vi "Pneumatic box control.vi"() -> ()   [LabVIEW 2018]
panel:
  out "出口气压":dbl(graph)
  out "x-y":u32
  out "错误输出 2":errorcluster caption="错误输出"
  out "手动给定值 4":dbl
  out "手动给定值 3":dbl
  out "手动给定值 2":dbl
  out "手动给定值":dbl
  in  "自动":bool=TRUE
  out "低负测量值":dbl
  out "低负给定值":dbl
  out "低正测量值":dbl
  out "低正给定值":dbl
  out "高负测量值":dbl
  out "高负给定值":dbl
  out "高正给定值":dbl
  out "高正测量值":dbl
  out "低负气压/psi":cluster{dbl, "低负":sgl}(graph)
  out "低正气压/psi":cluster{dbl, "低正":sgl}(graph)
  out "高负气压/psi":cluster{dbl, "高负":sgl}(graph)
  out "高正气压/psi":cluster{"高正":sgl, sgl}(graph)
  out "错误输出":errorcluster
  in  "case":dbl
  in  "停止":bool
  in  "低负":sgl(knob)=-0.22290154
  in  "高负":sgl(knob)=-1.1416342
  in  "低正":sgl(knob)=0.7104824 scale=0.0..2.0
  in  "高正":sgl(knob)=15.0 scale=0.0..15.0
  in  "低负开关":bool
  in  "低正开关":bool
  in  "大气压":bool
  in  "高负开关":bool
  in  "高正开关":bool
  in  "采样率":u32=255
  in  "DevIndex":i32
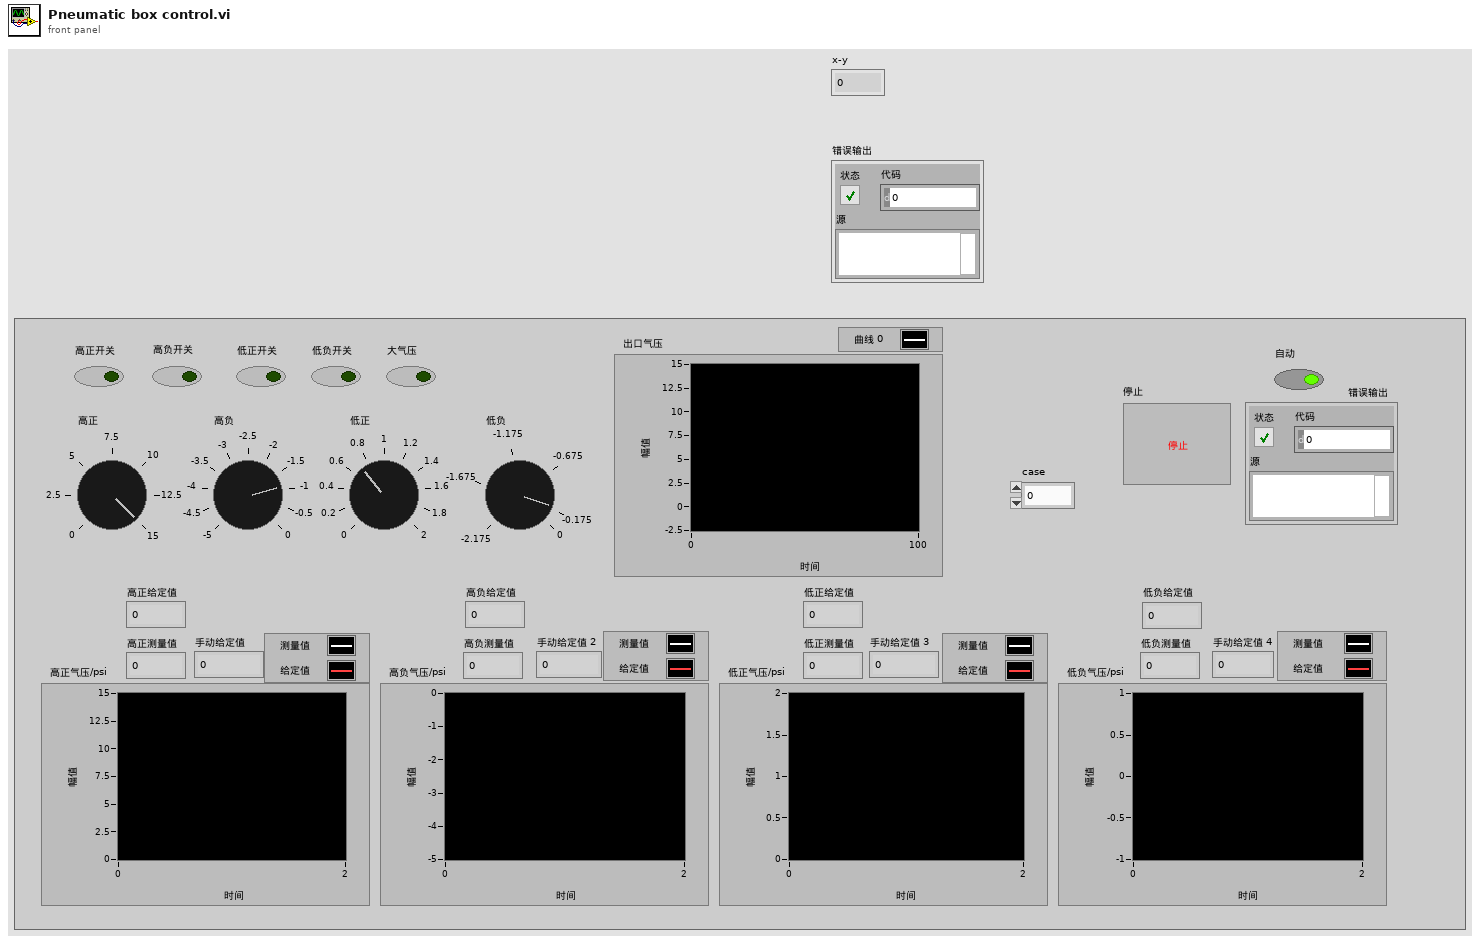
[diagram p1: front panel]
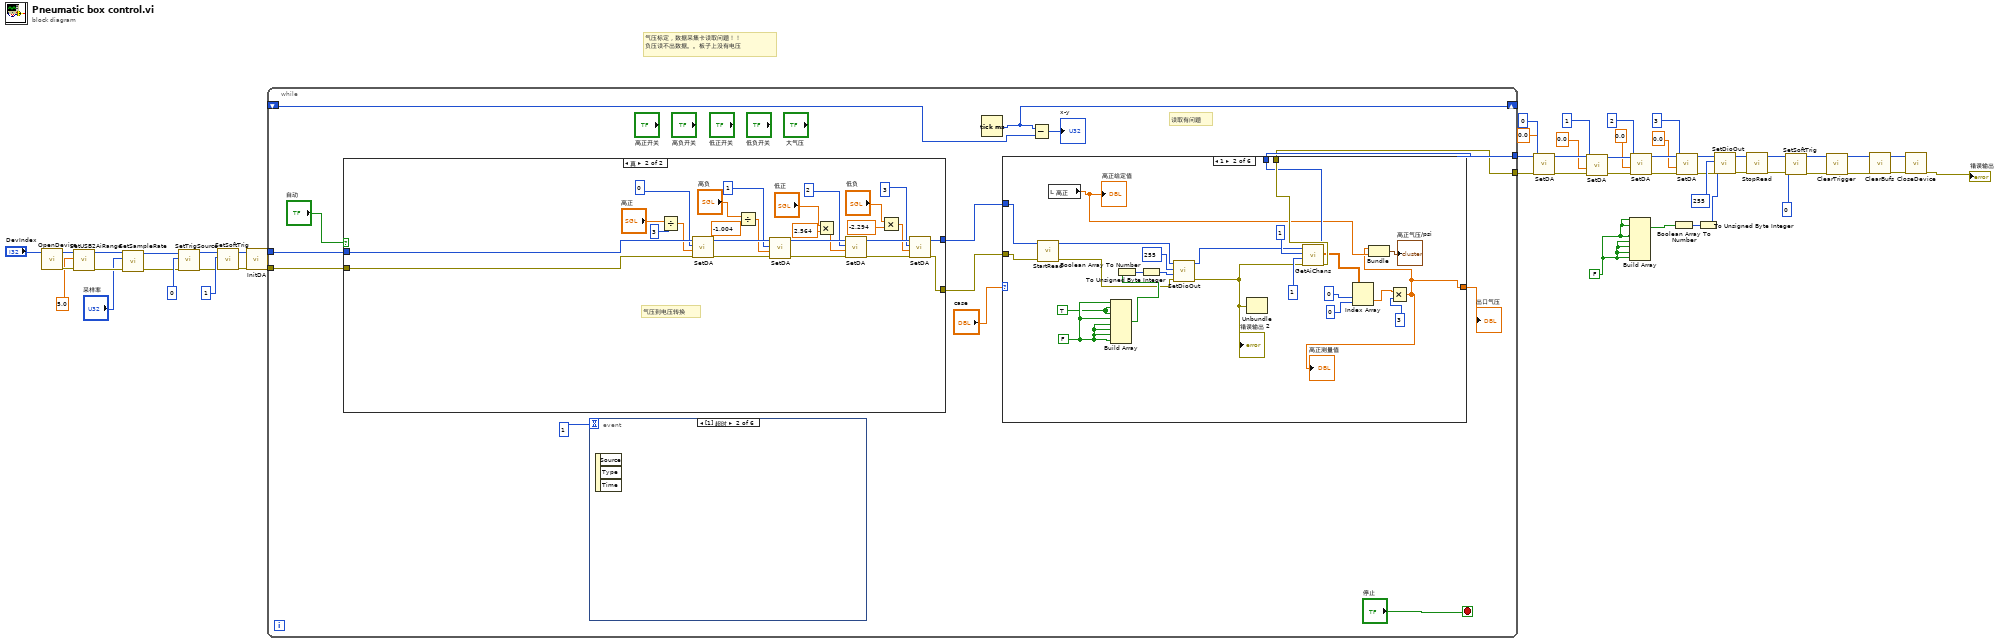
[diagram p0: block diagram]
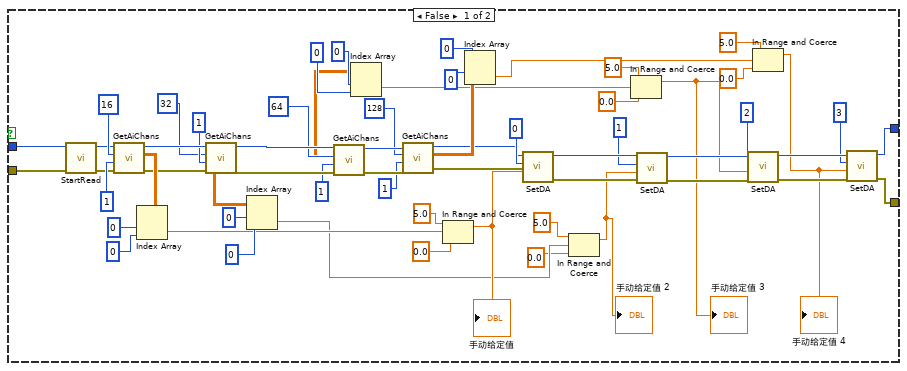
[diagram p2: hidden frame]
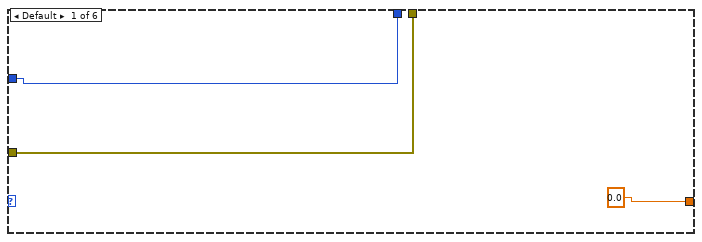
[diagram p3: hidden frame]
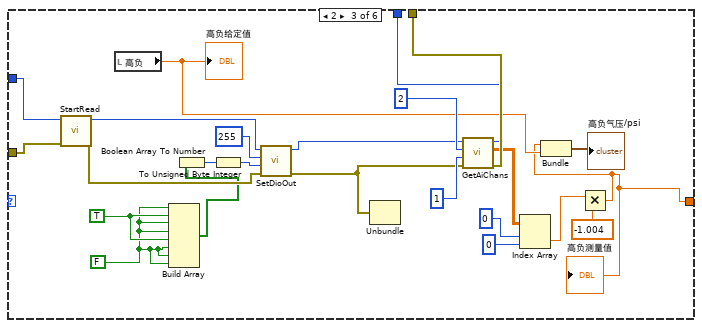
[diagram p4: hidden frame]
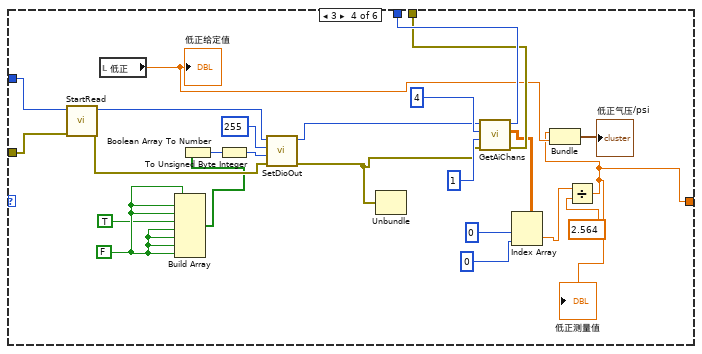
[diagram p5: hidden frame]
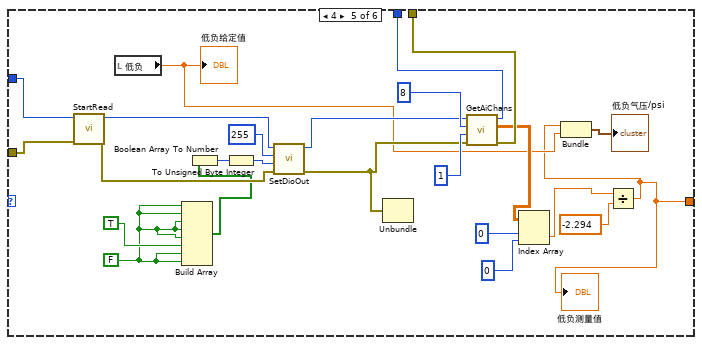
[diagram p6: hidden frame]
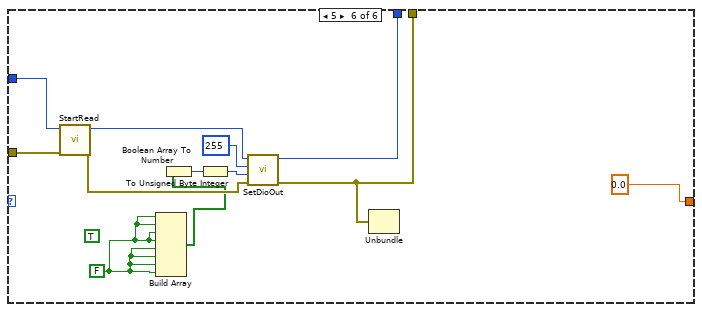
[diagram p7: hidden frame]
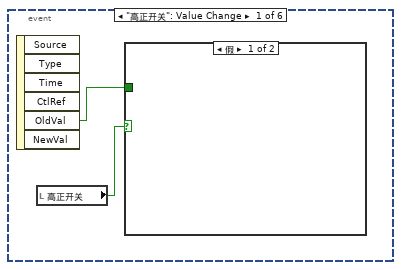
[diagram p8: hidden frame]
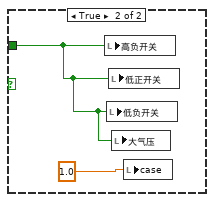
[diagram p9: hidden frame]
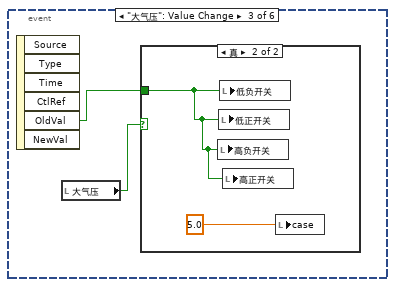
[diagram p10: hidden frame]
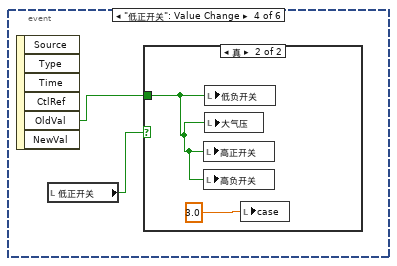
[diagram p12: hidden frame]
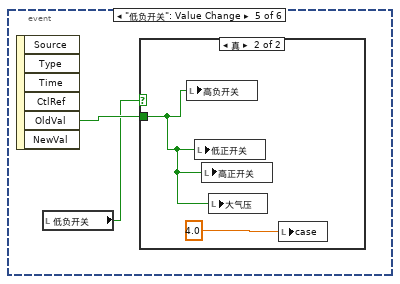
[diagram p14: hidden frame]
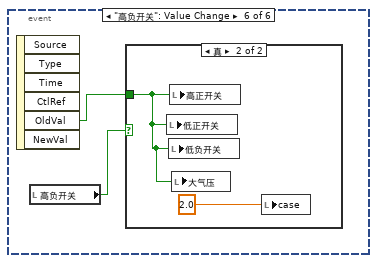
[diagram p16: hidden frame]
diagram:
  w9 = FALSE
  # "气压标定，数据采集卡读取问题！！\n负压读不出数据。。板子上没有电压"
  n1 = call "OpenDevice.vi"("DevIndex"="DevIndex") -> ("错误输出"=w44:errorcluster, "DevIndex Output"=w46:i32)  [unwired: 9 in]
  n2 = call "SetUSB2AiRange.vi"("错误输入（无错误）"=w44, "Range"=sgl 5.0, "DevIndex"=w46) -> ("错误输出"=w35:errorcluster, "DevIndex Output"=w37:i32)  [unwired: 7 in]
  n3 = call "SetSampleRate.vi"("错误输入（无错误）"=w35, "SampleRate"="采样率", "DevIndex"=w37) -> ("错误输出"=w34:errorcluster, "DevIndex Output"=w36:i32)  [unwired: 7 in]
  n4 = call "SetTrigSource.vi"("错误输入（无错误）"=w34, "TrigSource"=u8 0, "DevIndex"=w36) -> ("错误输出"=w39:errorcluster, "DevIndex Output"=w40:i32)  [unwired: 7 in]
  n5 = call "SetSoftTrig.vi"("错误输入（无错误）"=w39, "Trig"=u8 1, "DevIndex"=w40) -> ("错误输出"=w43:errorcluster, "DevIndex Output"=w45:i32)  [unwired: 7 in]
  n6 = call "InitDA.vi"("错误输入（无错误）"=w43, "DevIndex"=w45) -> ("错误输出"=w50:errorcluster, "DevIndex Output"=w51:i32)  [unwired: 8 in]
  n7 = while {
    tunnel: w51 -> [w65]
    tunnel: w50 -> [w64]
    tunnel: [w57] -> w11
    tunnel: [w56] -> w10
    shift-right: [w55] -> _
    shift-left: _ -> [w54]
    stop <- "停止" stop-if-true
    # "读取有问题"
    n8 = case shown="真" "自动" {
      tunnel: w65 -> [w116 w146]
      tunnel: w64 -> [w117 w145]
      tunnel: [w86 w141] -> w63
      tunnel: [w85 w140] -> w62
      frame False {
        n9 = call "StartRead.vi"("错误输入（无错误）"=w117, "DevIndex"=w116) -> ("错误输出"=w112:errorcluster, "DevIndex Output"=w114:i32)  [unwired: 8 in]
        n10 = call "GetAiChans.vi"("错误输入（无错误）"=w112, "Num"=u32 1, "ChanSel"=u16 16, "DevIndex"=w114) -> ("错误输出"=w102:errorcluster, "Ai"=w111:sgl[][], "DevIndex Output"=w103:i32)  [unwired: 4 in, 1 out]
        n11 = Index Array(array=w111, index (row)=0, index (col)=0) -> (element=w79:sgl)
        n12 = call "GetAiChans.vi"("错误输入（无错误）"=w102, "Num"=u32 1, "ChanSel"=u16 32, "DevIndex"=w103) -> ("错误输出"=w98:errorcluster, "Ai"=w108:sgl[][], "DevIndex Output"=w99:i32)  [unwired: 4 in, 1 out]
        n13 = Index Array(array=w108, index (row)=0, index (col)=0) -> (element=w78:sgl)
        n14 = call "GetAiChans.vi"("错误输入（无错误）"=w98, "Num"=u32 1, "ChanSel"=u16 64, "DevIndex"=w99) -> ("错误输出"=w93:errorcluster, "Ai"=w95:sgl[][], "DevIndex Output"=w94:i32)  [unwired: 4 in, 1 out]
        n15 = Index Array(array=w95, index (row)=0, index (col)=0) -> (element=w69:sgl)
        n16 = call "GetAiChans.vi"("错误输入（无错误）"=w93, "Num"=u32 1, "ChanSel"=u16 128, "DevIndex"=w94) -> ("错误输出"=w83:errorcluster, "Ai"=w90:sgl[][], "DevIndex Output"=w84:i32)  [unwired: 4 in, 1 out]
        n17 = In Range and Coerce(upper limit=5.0, x=w79, lower limit=0.0) -> (coerced(x)=w80:dbl)  [unwired: 1 out]
        "手动给定值" <- w80
        n18 = Index Array(array=w90, index (row)=0, index (col)=0) -> (element=w71:sgl)
        n19 = call "SetDA.vi"("错误输入（无错误）"=w83, "DAVolt"=w80, "DANum"=u8 0, "DevIndex"=w84) -> ("错误输出"=w125:errorcluster, "DevIndex Output"=w126:i32)  [unwired: 6 in]
        n20 = In Range and Coerce(upper limit=5.0, x=w78, lower limit=0.0) -> (coerced(x)=w67:dbl)  [unwired: 1 out]
        "手动给定值 2" <- w67
        n21 = In Range and Coerce(upper limit=5.0, x=w69, lower limit=0.0) -> (coerced(x)=w68:dbl)  [unwired: 1 out]
        "手动给定值 3" <- w68
        n22 = call "SetDA.vi"("错误输入（无错误）"=w125, "DAVolt"=w67, "DANum"=u8 1, "DevIndex"=w126) -> ("错误输出"=w124:errorcluster, "DevIndex Output"=w123:i32)  [unwired: 6 in]
        n23 = call "SetDA.vi"("错误输入（无错误）"=w124, "DAVolt"=w68, "DANum"=u8 2, "DevIndex"=w123) -> ("错误输出"=w121:errorcluster, "DevIndex Output"=w122:i32)  [unwired: 6 in]
        n24 = In Range and Coerce(upper limit=5.0, x=w71, lower limit=0.0) -> (coerced(x)=w70:dbl)  [unwired: 1 out]
        "手动给定值 4" <- w70
        n25 = call "SetDA.vi"("错误输入（无错误）"=w121, "DAVolt"=w70, "DANum"=u8 3, "DevIndex"=w122) -> ("错误输出"=w85:errorcluster, "DevIndex Output"=w86:i32)  [unwired: 6 in]
      }
      frame True {
        # "气压到电压转换"
        n26 = Divide(x="高正", y=3) -> (x/y=w130:sgl)
        n27 = call "SetDA.vi"("错误输入（无错误）"=w145, "DAVolt"=w130, "DANum"=u8 0, "DevIndex"=w146) -> ("错误输出"=w151:errorcluster, "DevIndex Output"=w152:i32)  [unwired: 6 in]
        n28 = Divide(x="高负", y=-1.004) -> (x/y=w128:dbl)
        n29 = call "SetDA.vi"("错误输入（无错误）"=w151, "DAVolt"=w128, "DANum"=u8 1, "DevIndex"=w152) -> ("错误输出"=w150:errorcluster, "DevIndex Output"=w149:i32)  [unwired: 6 in]
        n30 = Multiply(x="低正", y=2.564) -> (x*y=w129:dbl)
        n31 = call "SetDA.vi"("错误输入（无错误）"=w150, "DAVolt"=w129, "DANum"=u8 2, "DevIndex"=w149) -> ("错误输出"=w147:errorcluster, "DevIndex Output"=w148:i32)  [unwired: 6 in]
        n32 = Multiply(x="低负", y=-2.294) -> (x*y=w127:dbl)
        n33 = call "SetDA.vi"("错误输入（无错误）"=w147, "DAVolt"=w127, "DANum"=u8 3, "DevIndex"=w148) -> ("错误输出"=w140:errorcluster, "DevIndex Output"=w141:i32)  [unwired: 6 in]
      }
    }
    n34 = event shown="[1] 超时" {
      selector: _ -> [_ _ _ _ _ _]
      dyn-events: _ -> [_ _ _ _ _ _]
      timeout: 1 -> [_ _ _ _ _ _]
      event "高正开关": Value Change {
        n35 = event-data() -> ("OldVal"=w264:bool)  [unwired: 1 in, 5 out]
        n36 = local read "高正开关"() -> (w265:bool)
        n37 = case shown="假" w265 {
          tunnel: w264 -> [_ w267]
          frame False {
          }
          frame True {
            n38 = local write "高负开关"(w267) -> ()
            n39 = local write "低负开关"(w267) -> ()
            n40 = local write "低正开关"(w267) -> ()
            n41 = local write "大气压"(w267) -> ()
            n42 = local write "case"(1.0) -> ()
          }
        }
      }
      event Timeout {
        n43 = event-data() -> ()  [unwired: 1 in, 3 out]
      }
      event "大气压": Value Change {
        n44 = event-data() -> ("OldVal"=w268:bool)  [unwired: 1 in, 5 out]
        n45 = local read "大气压"() -> (w269:bool)
        n46 = case shown="真" w269 {
          tunnel: w268 -> [_ w271]
          frame False {
          }
          frame True {
            n47 = local write "高负开关"(w271) -> ()
            n48 = local write "低正开关"(w271) -> ()
            n49 = local write "低负开关"(w271) -> ()
            n50 = local write "高正开关"(w271) -> ()
            n51 = local write "case"(5.0) -> ()
          }
        }
      }
      event "低正开关": Value Change {
        n52 = event-data() -> ("OldVal"=w273:bool)  [unwired: 1 in, 5 out]
        n53 = local read "低正开关"() -> (w272:bool)
        n54 = case shown="真" w272 {
          tunnel: w273 -> [_ w275]
          frame False {
          }
          frame True {
            n55 = local write "高正开关"(w275) -> ()
            n56 = local write "高负开关"(w275) -> ()
            n57 = local write "低负开关"(w275) -> ()
            n58 = local write "大气压"(w275) -> ()
            n59 = local write "case"(3.0) -> ()
          }
        }
      }
      event "低负开关": Value Change {
        n60 = event-data() -> ("OldVal"=w277:bool)  [unwired: 1 in, 5 out]
        n61 = local read "低负开关"() -> (w276:bool)
        n62 = case shown="真" w276 {
          tunnel: w277 -> [_ w279]
          frame False {
          }
          frame True {
            n63 = local write "高负开关"(w279) -> ()
            n64 = local write "低正开关"(w279) -> ()
            n65 = local write "高正开关"(w279) -> ()
            n66 = local write "大气压"(w279) -> ()
            n67 = local write "case"(4.0) -> ()
          }
        }
      }
      event "高负开关": Value Change {
        n68 = event-data() -> ("OldVal"=w281:bool)  [unwired: 1 in, 5 out]
        n69 = local read "高负开关"() -> (w280:bool)
        n70 = case shown="真" w280 {
          tunnel: w281 -> [_ w283]
          frame False {
          }
          frame True {
            n71 = local write "低正开关"(w283) -> ()
            n72 = local write "低负开关"(w283) -> ()
            n73 = local write "高正开关"(w283) -> ()
            n74 = local write "大气压"(w283) -> ()
            n75 = local write "case"(2.0) -> ()
          }
        }
      }
    }
    n76 = Tick Count (ms)() -> (millisecond timer value=w55:u32)
    n77 = case shown="1" "case" {
      tunnel: w63 -> [w155 w175 w197 w221 w245 w257]
      tunnel: w62 -> [w154 w174 w196 w220 w244 w256]
      tunnel: [w155 w164 w188 w215 w237 w254] -> w57
      tunnel: [w154 w165 w189 w214 w238 w253] -> w56
      tunnel: [0.0 w156 w180 w206 w229 0.0] -> w60
      frame Default {
      }
      frame 1 {
        w172 = TRUE
        w173 = FALSE
        n78 = call "StartRead.vi"("错误输入（无错误）"=w174, "DevIndex"=w175) -> ("错误输出"=w170:errorcluster, "DevIndex Output"=w171:i32)  [unwired: 8 in]
        n79 = local read "高正"() -> (w159:sgl)
        "高正给定值" <- w159
        n80 = Build Array(w173, w172, w172, w173, w173, w173, w173, w173) -> (w176:bool[])
        n81 = Boolean Array To Number(Boolean array=w176) -> (number=w179:u32)
        n82 = To Unsigned Byte Integer(number=w179) -> (unsigned 8bit integer=w178:u8)
        n83 = call "SetDioOut.vi"("错误输入（无错误）"=w170, "DioOut"=w178, "DioChanSel"=u8 255, "DevIndex"=w171) -> ("错误输出"=w166:errorcluster, "DevIndex Output"=w167:i32)  [unwired: 6 in]
        "错误输出 2" <- w166
        n84 = Unbundle(w166) -> ()  [unwired: 3 out]
        n85 = call "GetAiChans.vi"("错误输入（无错误）"=w166, "Num"=u32 1, "ChanSel"=u16 1, "DevIndex"=w167) -> ("错误输出"=w165:errorcluster, "Ai"=w161:sgl[][], "DevIndex Output"=w164:i32)  [unwired: 4 in, 1 out]
        n86 = Index Array(array=w161, index (row)=0, index (col)=0) -> (element=w157:sgl)
        n87 = Multiply(x=w157, y=3) -> (x*y=w156:sgl)
        "高正测量值" <- w156
        n88 = Bundle(w156, "高正"=w159) -> (→"高正气压/psi":cluster{sgl, "高正":sgl})  [unwired: 1 in]
      }
      frame 2 {
        w195 = TRUE
        w194 = FALSE
        n89 = call "StartRead.vi"("错误输入（无错误）"=w196, "DevIndex"=w197) -> ("错误输出"=w199:errorcluster, "DevIndex Output"=w200:i32)  [unwired: 8 in]
        n90 = local read "高负"() -> (w184:sgl)
        "高负给定值" <- w184
        n91 = Build Array(w194, w195, w194, w194, w195, w194, w194, w194) -> (w198:bool[])
        n92 = Boolean Array To Number(Boolean array=w198) -> (number=w203:u32)
        n93 = To Unsigned Byte Integer(number=w203) -> (unsigned 8bit integer=w202:u8)
        n94 = call "SetDioOut.vi"("错误输入（无错误）"=w199, "DioOut"=w202, "DioChanSel"=u8 255, "DevIndex"=w200) -> ("错误输出"=w190:errorcluster, "DevIndex Output"=w191:i32)  [unwired: 6 in]
        n95 = Unbundle(w190) -> ()  [unwired: 3 out]
        n96 = call "GetAiChans.vi"("错误输入（无错误）"=w190, "Num"=u32 1, "ChanSel"=u16 2, "DevIndex"=w191) -> ("错误输出"=w189:errorcluster, "Ai"=w185:sgl[][], "DevIndex Output"=w188:i32)  [unwired: 4 in, 1 out]
        n97 = Index Array(array=w185, index (row)=0, index (col)=0) -> (element=w182:sgl)
        n98 = Multiply(x=w182, y=-1.004) -> (x*y=w180:dbl)
        "高负测量值" <- w180
        n99 = Bundle(w180, "高负"=w184) -> (→"高负气压/psi":cluster{dbl, "高负":sgl})  [unwired: 1 in]
      }
      frame 3 {
        w205 = FALSE
        n100 = call "StartRead.vi"("错误输入（无错误）"=w220, "DevIndex"=w221) -> ("错误输出"=w223:errorcluster, "DevIndex Output"=w224:i32)  [unwired: 8 in]
        n101 = local read "低正"() -> (w209:sgl)
        "低正给定值" <- w209
        n102 = Build Array(w205, w205, w205, TRUE, w205, w205, w205, w205) -> (w222:bool[])
        n103 = Boolean Array To Number(Boolean array=w222) -> (number=w227:u32)
        n104 = To Unsigned Byte Integer(number=w227) -> (unsigned 8bit integer=w226:u8)
        n105 = call "SetDioOut.vi"("错误输入（无错误）"=w223, "DioOut"=w226, "DioChanSel"=u8 255, "DevIndex"=w224) -> ("错误输出"=w216:errorcluster, "DevIndex Output"=w217:i32)  [unwired: 6 in]
        n106 = Unbundle(w216) -> ()  [unwired: 3 out]
        n107 = call "GetAiChans.vi"("错误输入（无错误）"=w216, "Num"=u32 1, "ChanSel"=u16 4, "DevIndex"=w217) -> ("错误输出"=w214:errorcluster, "Ai"=w211:sgl[][], "DevIndex Output"=w215:i32)  [unwired: 4 in, 1 out]
        n108 = Index Array(array=w211, index (row)=0, index (col)=0) -> (element=w208:sgl)
        n109 = Divide(x=w208, y=2.564) -> (x/y=w206:dbl)
        "低正测量值" <- w206
        n110 = Bundle(w206, "低正"=w209) -> (→"低正气压/psi":cluster{dbl, "低正":sgl})  [unwired: 1 in]
      }
      frame 4 {
        w228 = FALSE
        n111 = call "StartRead.vi"("错误输入（无错误）"=w244, "DevIndex"=w245) -> ("错误输出"=w247:errorcluster, "DevIndex Output"=w248:i32)  [unwired: 8 in]
        n112 = local read "低负"() -> (w233:sgl)
        "低负给定值" <- w233
        n113 = Build Array(w228, w228, w228, w228, w228, TRUE, w228, w228) -> (w246:bool[])
        n114 = Boolean Array To Number(Boolean array=w246) -> (number=w251:u32)
        n115 = To Unsigned Byte Integer(number=w251) -> (unsigned 8bit integer=w250:u8)
        n116 = call "SetDioOut.vi"("错误输入（无错误）"=w247, "DioOut"=w250, "DioChanSel"=u8 255, "DevIndex"=w248) -> ("错误输出"=w239:errorcluster, "DevIndex Output"=w240:i32)  [unwired: 6 in]
        n117 = Unbundle(w239) -> ()  [unwired: 3 out]
        n118 = call "GetAiChans.vi"("错误输入（无错误）"=w239, "Num"=u32 1, "ChanSel"=u16 8, "DevIndex"=w240) -> ("错误输出"=w238:errorcluster, "Ai"=w234:sgl[][], "DevIndex Output"=w237:i32)  [unwired: 4 in, 1 out]
        n119 = Index Array(array=w234, index (row)=0, index (col)=0) -> (element=w231:sgl)
        n120 = Divide(x=w231, y=-2.294) -> (x/y=w229:dbl)
        "低负测量值" <- w229
        n121 = Bundle(w229, "低负"=w233) -> (→"低负气压/psi":cluster{dbl, "低负":sgl})  [unwired: 1 in]
      }
      frame 5 {
        (unwired) TRUE
        w255 = FALSE
        n122 = call "StartRead.vi"("错误输入（无错误）"=w256, "DevIndex"=w257) -> ("错误输出"=w259:errorcluster, "DevIndex Output"=w260:i32)  [unwired: 8 in]
        n123 = Build Array(w255, w255, w255, w255, w255, w255, w255, w255) -> (w258:bool[])
        n124 = Boolean Array To Number(Boolean array=w258) -> (number=w263:u32)
        n125 = To Unsigned Byte Integer(number=w263) -> (unsigned 8bit integer=w262:u8)
        n126 = call "SetDioOut.vi"("错误输入（无错误）"=w259, "DioOut"=w262, "DioChanSel"=u8 255, "DevIndex"=w260) -> ("错误输出"=w253:errorcluster, "DevIndex Output"=w254:i32)  [unwired: 6 in]
        n127 = Unbundle(w253) -> ()  [unwired: 3 out]
      }
    }
    "出口气压" <- w60
    n128 = Subtract(x=w55, y=w54) -> (x-y=→"x-y":u32)
  }
  n129 = call "SetDA.vi"("错误输入（无错误）"=w10, "DAVolt"=0.0, "DANum"=u8 0, "DevIndex"=w11) -> ("错误输出"=w24:errorcluster, "DevIndex Output"=w25:i32)  [unwired: 6 in]
  n130 = call "SetDA.vi"("错误输入（无错误）"=w24, "DAVolt"=0.0, "DANum"=u8 1, "DevIndex"=w25) -> ("错误输出"=w23:errorcluster, "DevIndex Output"=w22:i32)  [unwired: 6 in]
  n131 = Build Array(w9, w9, w9, w9, w9, w9, w9, w9) -> (w7:bool[])
  n132 = call "SetDA.vi"("错误输入（无错误）"=w23, "DAVolt"=0.0, "DANum"=u8 2, "DevIndex"=w22) -> ("错误输出"=w20:errorcluster, "DevIndex Output"=w21:i32)  [unwired: 6 in]
  n133 = Boolean Array To Number(Boolean array=w7) -> (number=w8:u32)
  n134 = call "SetDA.vi"("错误输入（无错误）"=w20, "DAVolt"=0.0, "DANum"=u8 3, "DevIndex"=w21) -> ("错误输出"=w3:errorcluster, "DevIndex Output"=w4:i32)  [unwired: 6 in]
  n135 = To Unsigned Byte Integer(number=w8) -> (unsigned 8bit integer=w6:u8)
  n136 = call "SetDioOut.vi"("错误输入（无错误）"=w3, "DioOut"=w6, "DioChanSel"=u8 255, "DevIndex"=w4) -> ("错误输出"=w2:errorcluster, "DevIndex Output"=w1:i32)  [unwired: 6 in]
  n137 = call "StopRead.vi"("错误输入（无错误）"=w2, "DevIndex"=w1) -> ("错误输出"=w31:errorcluster, "DevIndex Output"=w32:i32)  [unwired: 8 in]
  n138 = call "SetSoftTrig.vi"("错误输入（无错误）"=w31, "Trig"=u8 0, "DevIndex"=w32) -> ("错误输出"=w30:errorcluster, "DevIndex Output"=w28:i32)  [unwired: 7 in]
  n139 = call "ClearTrigger.vi"("错误输入（无错误）"=w30, "DevIndex"=w28) -> ("错误输出"=w29:errorcluster, "DevIndex Output"=w27:i32)  [unwired: 8 in]
  n140 = call "ClearBufs.vi"("错误输入（无错误）"=w29, "DevIndex"=w27) -> ("错误输出"=w47:errorcluster, "DevIndex Output"=w48:i32)  [unwired: 8 in]
  n141 = call "CloseDevice.vi"("错误输入（无错误）"=w47, "DevIndex"=w48) -> ("错误输出"=→"错误输出":errorcluster)  [unwired: 8 in, 1 out]
